vi "DoScaleCalibration.vi"(8 "Error In":errorcluster, 10 "TLCamera reference in":refnum<k24>, 11 "MotorController in":refnum<class "MotorController.lvclass">) -> (0 "Error Out":errorcluster, 2 "TLCamera reference out":refnum<k24>, 3 "MotorController out":refnum<class "MotorController.lvclass">)   [LabVIEW 2019]
uses:
  MotorController.lvclass
  C:/Users/jleeman/git_repos/CAxis_Machine/C-Axis LabView Controller/Library_X64/Thorlabs.TSI.TLCameraInterfaces.dll
  Library_X64/Thorlabs.TSI.TLCameraInterfaces.dll
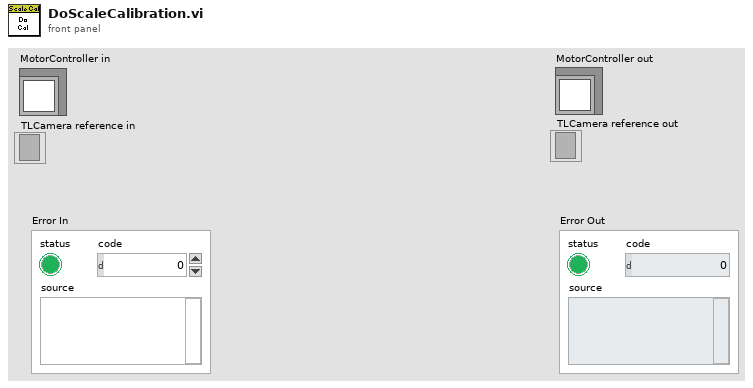
[diagram p1: front panel]
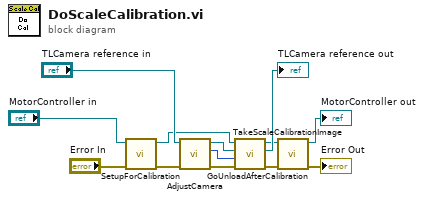
[diagram p0: block diagram]
diagram:
  n1 = call "SetupForCalibration.vi"("Error In"="Error In", "MotorController in"="MotorController in") -> ("Error Out"=w1:errorcluster, "MotorController out"=w4:refnum<class "MotorController.lvclass">)  [unwired: 8 in]
  n2 = call "AdjustCamera.vi"("Error In"=w1, "TLCamera reference in"="TLCamera reference in") -> ("Error Out"=w10:errorcluster, "Exposure (us)"=w11:u32, "TLCamera reference out"=w12:refnum<k24>)  [unwired: 7 in]
  n3 = call "TakeScaleCalibrationImage.vi"("Error In"=w10, "ExposureTime_us"=w11, "TLCamera reference in"=w12, "MotorController in"=w4) -> ("Error Out"=w6:errorcluster, "TLCamera reference out"=→"TLCamera reference out":refnum<k24>, "MotorController out"=w5:refnum<class "MotorController.lvclass">)  [unwired: 5 in]
  n4 = call "GoUnloadAfterCalibration.vi"("Error In"=w6, "MotorController in"=w5) -> ("Error Out"=→"Error Out":errorcluster, "MotorController out"=→"MotorController out":refnum<class "MotorController.lvclass">)  [unwired: 8 in]
